vi "Image Process.vi"(7 "Particle Measurements (Pixels)":dbl[][](array[numeric])=[[126.4410480349345, 189.5240174672489], [176.61198428290766, 196.4106090373281], [77.19657142857143, 196.89371428571428]] format="%.2f", 8 "Vision PID gains":T1={"proportional gain (Kc)"=0.003, "integral time (Ti, min)"=0.0, "derivative time (Td, min)"=0.0} {"derivative time (Td, min)" format="%.3f"; "integral time (Ti, min)" format="%.3f"; "proportional gain (Kc)" format="%.3f"}) -> (0 "A":dbl=-0.0364106090373281, 2 "String":string="-0.036411,-0.036411")   [LabVIEW 2012]
uses:
  <vilib>/addons/control/pid/pid.llb/PID (DBL).vi
  <vilib>/addons/control/pid/NI_PID_pid.lvlib
panel:
  out "C":dbl format="%.2f"
  out "B":dbl=-0.0364106090373281
  in  "Vision PID limits":cluster{"output high":dbl, "output low":dbl}={"output high"=1.0, "output low"=-1.0} {"output low" format="%.2f"; "output high" format="%.2f"}
  # "P= 0.003\nI = 0\nD = 0"
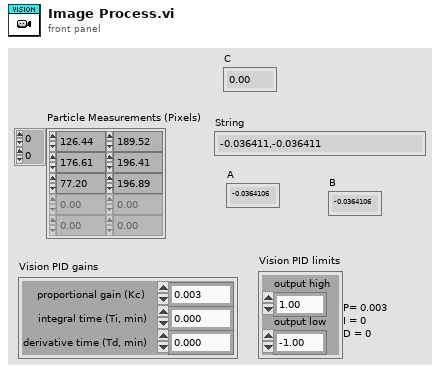
[diagram p1: front panel]
types:
  T1 = cluster{"proportional gain (Kc)":dbl, "integral time (Ti, min)":dbl, "derivative time (Td, min)":dbl}
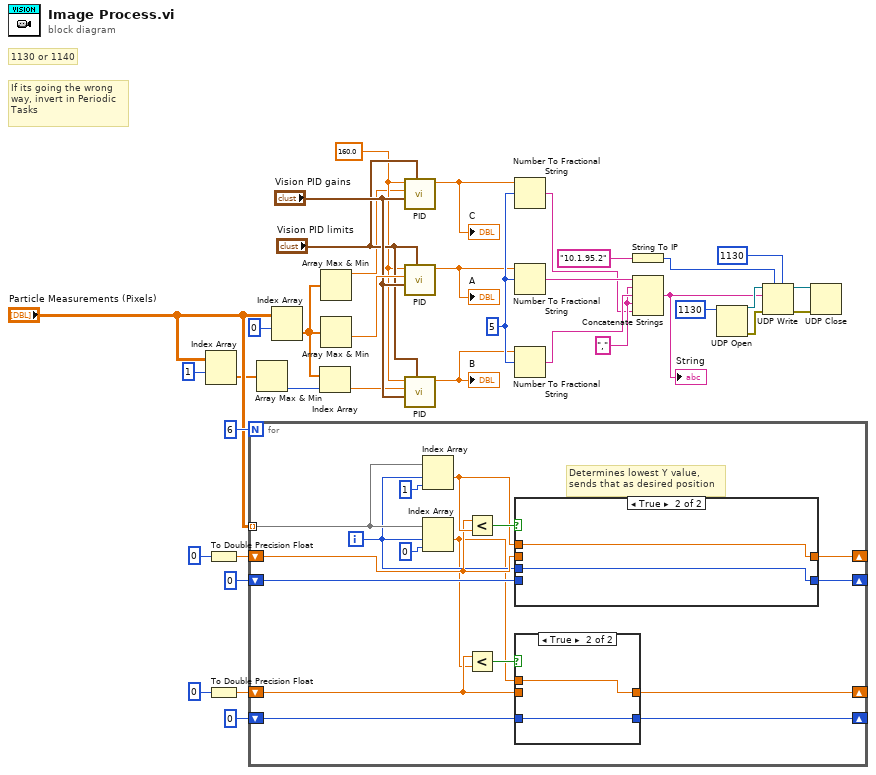
[diagram p0: block diagram]
diagram:
  w9 = i16 5 ("width (-)")
  w10 = "," ("string")
  w12 = 160.0 ("setpoint")
  # "If its going the wrong\nway, invert in Periodic\nTasks"
  # "1130 or 1140"
  n1 = Index Array(array="Particle Measurements (Pixels)", index (row)=1) -> (element=w7:dbl[])  [unwired: 1 in]
  n2 = To Double Precision Float(number=0) -> (double precision float=w26:dbl)
  n3 = To Double Precision Float(number=0) -> (double precision float=w21:dbl)
  n4 = for {
    N: 6 -> [_]
    tunnel: "Particle Measurements (Pixels)" -> [w44] mode=indexing
    shift-right: [w50] -> _
    shift-left: w26 -> [w46]
    shift-right: [w49] -> _
    shift-left: 0 -> [w51]
    shift-right: [w37] -> _
    shift-left: w21 -> [w39]
    shift-right: [w41] -> _
    shift-left: 0 ("index") -> [w42]
    i -> [w43]
    # "Determines lowest Y value,\nsends that as desired position"
    n5 = Index Array(array=w44, index #1=w43, index #2=1 ("disabled index (col)")) -> (element #1=w47:dbl)  [unwired: 1 out]
    n6 = Index Array(array=w44, index #1=w43, index #2=0 ("index")) -> (element #1=w38:dbl)  [unwired: 1 out]
    n7 = Less?(x=w46, y=w47) -> (x < y?=w52:bool)
    n8 = Less?(x=w39, y=w38) -> (x < y?=w40:bool)
    n9 = case shown="True" w52 {
      tunnel: w43 -> [_ w60]
      tunnel: [w57 w60] -> w49
      tunnel: w47 -> [_ w59]
      tunnel: [w58 w59] -> w50
      tunnel: w46 -> [w58 _]
      tunnel: w51 -> [w57 _]
      frame False {
      }
      frame True {
      }
    }
    n10 = case shown="True" w40 {
      tunnel: w42 -> [w53 w56]
      tunnel: [w53 w56] -> w41
      tunnel: w39 -> [w54 _]
      tunnel: w38 -> [_ w55]
      tunnel: [w54 w55] -> w37
      frame False {
      }
      frame True {
      }
    }
  }
  n11 = Array Max & Min(array=w7) -> (min index (indices)=w6:i32)  [unwired: 3 out]
  n12 = Index Array(array="Particle Measurements (Pixels)", index (row)=0) -> (element=w5:dbl[])  [unwired: 1 in]
  n13 = Index Array(array=w5, index=w6) -> (element=w4:dbl)
  n14 = Array Max & Min(array=w5) -> (max value=w11:dbl)  [unwired: 3 out]
  n15 = Array Max & Min(array=w5) -> (min value=w15:dbl)  [unwired: 3 out]
  n16 = call-poly <vilib>:"PID.vi"("output range"="Vision PID limits", "PID gains"="Vision PID gains", "process variable"=w11, "setpoint"=w12) -> ("output"=w2:dbl)  [unwired: 6 in, 1 out]
  "C" <- w2
  n17 = call-poly <vilib>:"PID.vi"("output range"="Vision PID limits", "PID gains"="Vision PID gains", "process variable"=w15, "setpoint"=w12) -> ("output"=w3:dbl)  [unwired: 6 in, 1 out]
  "A" <- w3
  n18 = call-poly <vilib>:"PID.vi"("output range"="Vision PID limits", "PID gains"="Vision PID gains", "process variable"=w4, "setpoint"=w12) -> ("output"=w1:dbl)  [unwired: 6 in, 1 out]
  "B" <- w1
  n19 = Number To Fractional String(number=w2, width (-)=w9) -> (F-format string=w8:string)  [unwired: 2 in]
  n20 = Number To Fractional String(number=w3, width (-)=w9) -> (F-format string=w23:string)  [unwired: 2 in]
  n21 = Number To Fractional String(number=w1, width (-)=w9) -> (F-format string=w19:string)  [unwired: 2 in]
  n22 = String To IP(1:"10.1.95.2" ("name")) -> (0:w30:u32)
  n23 = Concatenate Strings(w23, w10, w19, w10, w8) -> (w24:string)
  "String" <- w24
  n24 = UDP Open(11:u16 1130 ("port")) -> (port=w35:refnum<k16>, 0:w34:errorcluster)  [unwired: 4 in, 1 out]
  n25 = UDP Write(address=w30, port or service name=u16 1130, connection ID=w35, data in=w24, 8:w34) -> (error out=w33:errorcluster, 3:w32:refnum<k16>)  [unwired: 1 in]
  n26 = UDP Close(connection ID=w32, 8:w33) -> ()  [unwired: 2 out]
